vi "saveItems.vi"(8 "error in (no error)":errorcluster, 11 "Array":T1[](array[typedef])) -> (0 "error out":errorcluster)   [LabVIEW 2021]
uses:
  Item.ctl
  <vilib>/Utility/config.llb/Write Key (String).vi
  <vilib>/Utility/config.llb/Write Key (Double).vi
  <vilib>/Utility/config.llb/NI_LVConfig.lvlib
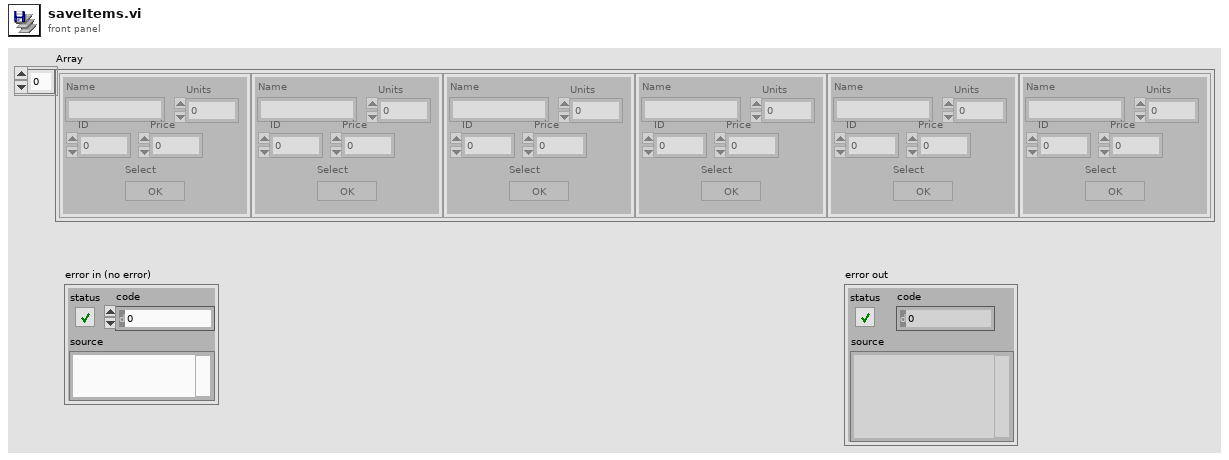
[diagram p1: front panel]
types:
  T1 = typedef "Item.ctl" = cluster{"Name":string, "ID":dbl, "Price":dbl, "Select":bool, "Units":dbl}
  T2 = typedef "NI_LVConfig.lvlib/Config Data RefNum.ctl" = refnum<k1>
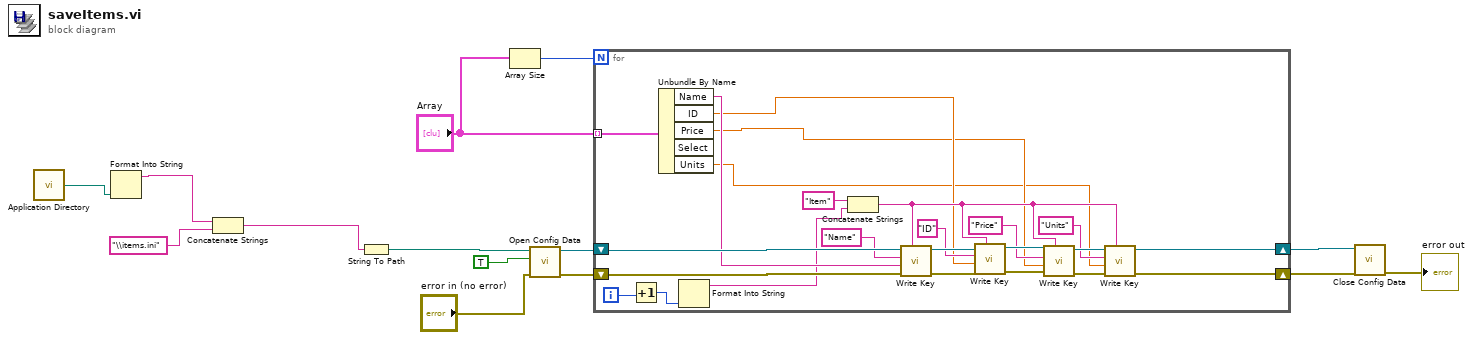
[diagram p0: block diagram]
diagram:
  n1 = call <vilib>:"Application Directory.vi"() -> ("Application Directory"=w5:path)
  n2 = Format Into String(w5) -> (resulting string=w4:string)  [unwired: 3 in, 1 out]
  n3 = Concatenate Strings(w4, "\\items.ini" ("string")) -> (w2:string)
  n4 = String To Path(string=w2) -> (path=w1:path)
  n5 = Array Size(array="Array") -> (size(s)=w14:i32)
  n6 = call <vilib>:"Open Config Data.vi"("error in (no error)"="error in (no error)", "create file if necessary (T)"=TRUE, "configuration file path"=w1) -> ("error out"=w10:errorcluster, "refnum"=w11:T2)  [unwired: 6 in, 1 out]
  n7 = for {
    N: w14 -> [_]
    tunnel: "Array" -> [w38] mode=indexing
    shift-right: [w32] -> w8
    shift-left: w10 -> [w36]
    shift-right: [w28] -> w9
    shift-left: w11 -> [w37]
    i -> [w16]
    n8 = Increment(x=w16) -> (x+1=w15:i32)
    n9 = Unbundle By Name(w38) -> ("Name"=w27:string, "ID"=w19:dbl, "Price"=w18:dbl, "Units"=w17:dbl)  [unwired: 1 out]
    n10 = Format Into String(w15) -> (resulting string=w21:string)  [unwired: 3 in, 1 out]
    n11 = Concatenate Strings("Item" ("section"), w21) -> (w20:string)
    n12 = call-poly <vilib>:"Write Key.vi"("section"=w20, "error in (no error)"=w36, "value"=w27, "key"="Name", "refnum"=w37) -> ("error out"=w35:errorcluster, "refnum out"=w31:T2)  [unwired: 4 in, 1 out]
    n13 = call-poly <vilib>:"Write Key.vi"("section"=w20, "error in (no error)"=w35, "value"=w19, "key"="ID", "refnum"=w31) -> ("error out"=w34:errorcluster, "refnum out"=w30:T2)  [unwired: 4 in, 1 out]
    n14 = call-poly <vilib>:"Write Key.vi"("section"=w20, "error in (no error)"=w34, "value"=w18, "key"="Price", "refnum"=w30) -> ("error out"=w33:errorcluster, "refnum out"=w29:T2)  [unwired: 4 in, 1 out]
    n15 = call-poly <vilib>:"Write Key.vi"("section"=w20, "error in (no error)"=w33, "value"=w17, "key"="Units", "refnum"=w29) -> ("error out"=w32:errorcluster, "refnum out"=w28:T2)  [unwired: 4 in, 1 out]
  }
  n16 = call <vilib>:"Close Config Data.vi"("error in (no error)"=w8, "refnum"=w9) -> ("error out"=→"error out":errorcluster)  [unwired: 8 in, 1 out]
